vi "AlliGator Save SGL Gate Image to HDF5.vi"(6 "Compression":bool, 7 "Replace?":bool, 8 "error in (no error)":errorcluster, 9 "Image Name":string, 10 "Data":sgl[][](array[numeric]), 11 "ref in":T1 format="%.0x") -> (0 "error out":errorcluster, 3 "ref out":T1 format="%.0x")   [LabVIEW 2021, in "AlliGator Files.lvlib"]
doc: "Saves single gate image data array to HDF5 FLI Dataset file."
uses:
  AlliGator Files.lvlib
  <vilib>/addons/h5labview2/base/hid_t.ctl
  <vilib>/addons/h5labview2/base/lib_path.vi
  <vilib>/addons/h5labview2/base/H5Equery.vi
  <vilib>/addons/h5labview2/dataset/H5Dwrite.llb/H5Dwrite.xnode
  <vilib>/addons/h5labview2/props/H5P.lvlib
  <vilib>/addons/h5labview2/space/H5S.lvlib
  <vilib>/addons/h5labview2/type/H5T.lvlib
  <vilib>/addons/h5labview2/dataset/H5D.lvlib
panel:
  # "see the AlliGator License on the block diagram (Ctrl+E or Window:Show Block Diagram)"
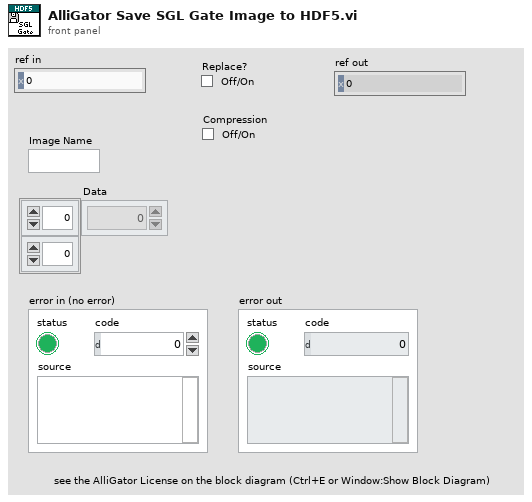
[diagram p1: front panel]
types:
  T1 = typedef "hid_t.ctl" = i64
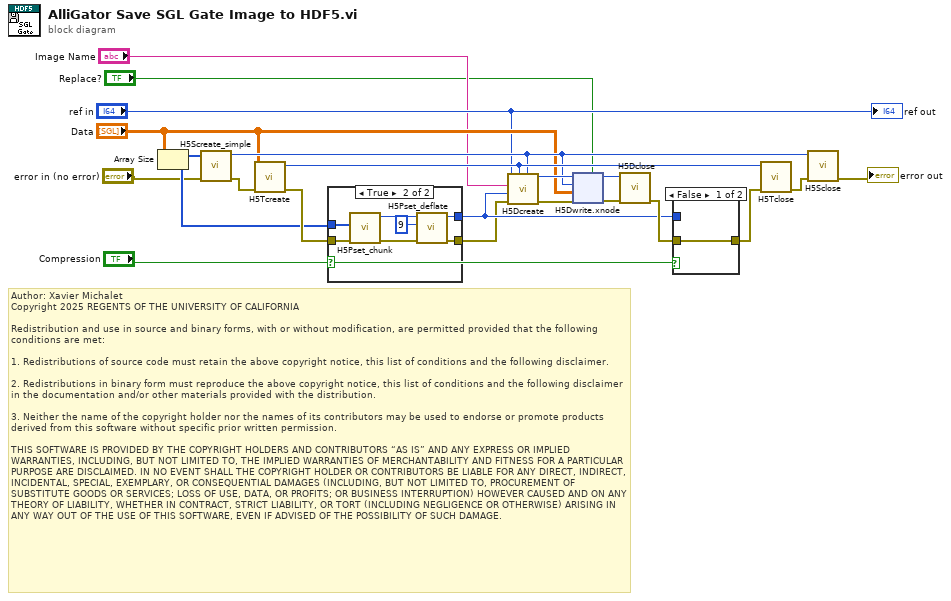
[diagram p0: block diagram]
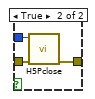
[diagram p2: hidden frame]
diagram:
  # "Author: Xavier Michalet\nCopyright 2025 REGENTS OF THE UNIVERSITY OF CALIFORNIA\n\nRedistribution and use in source and binary forms, with or without modification, are permitted provided that the following conditions are met:\n\n1. Redistributions of source code must retain the above copyright notice, this list of conditions and the following disclaimer.\n\n2. Redistributions in binary form must reproduce the above copyright notice, this list of conditions and the following disclaimer in the documentation and/or other materials provided with the distribution.\n\n3. Neither the name of the copyright holder nor the names of its contributors may be used to endorse or promote products derived from this software without specific prior written permission.\n\nTHIS SOFTWARE IS PROVIDED BY THE COPYRIGHT HOLDERS AND CONTRIBUTORS “AS IS” AND ANY EXPRESS OR IMPLIED WARRANTIES, INCLUDING, BUT NOT LIMITED TO, THE IMPLIED WARRANTIES OF MERCHANTABILITY AND FITNESS FOR A PARTICULAR PURPOSE ARE DISCLAIMED. IN NO EVENT SHALL THE COPYRIGHT HOLDER OR CONTRIBUTORS BE LIABLE FOR ANY DIRECT, INDIRECT, INCIDENTAL, SPECIAL, EXEMPLARY, OR CONSEQUENTIAL DAMAGES (INCLUDING, BUT NOT LIMITED TO, PROCUREMENT OF SUBSTITUTE GOODS OR SERVICES; LOSS OF USE, DATA, OR PROFITS; OR BUSINESS INTERRUPTION) HOWEVER CAUSED AND ON ANY THEORY OF LIABILITY, WHETHER IN CONTRACT, STRICT LIABILITY, OR TORT (INCLUDING NEGLIGENCE OR OTHERWISE) ARISING IN ANY WAY OUT OF THE USE OF THIS SOFTWARE, EVEN IF ADVISED OF THE POSSIBILITY OF SUCH DAMAGE."
  n1 = Array Size(array="Data") -> (size(s)=w8:i32[])
  n2 = call <vilib>:"H5Screate_simple.vi"("error in (no error)"="error in (no error)", "dims"=w8) -> ("error out"=w17:errorcluster, "space out"=w10:T1)  [unwired: 7 in, 1 out]
  n3 = call <vilib>:"H5Tcreate.vi"("error in (no error)"=w17, "type variant"="Data") -> ("error out"=w16:errorcluster, "type out"=w13:T1)  [unwired: 7 in, 1 out]
  n4 = case shown="True" "Compression" {
    tunnel: w16 -> [w22 w29]
    tunnel: [_ w28] -> w11
    tunnel: [w22 w24] -> w9
    tunnel: w8 -> [_ w23]
    frame False {
    }
    frame True {
      n5 = call <vilib>:"H5Pset_chunk.vi"("error in (no error)"=w29, "chunk size"=w23) -> ("error out"=w26:errorcluster, "prop out"=w27:T1)  [unwired: 8 in]
      n6 = call <vilib>:"H5Pset_deflate.vi"("error in (no error)"=w26, "level"=u8 9, "prop in"=w27) -> ("error out"=w24:errorcluster, "prop out"=w28:T1)  [unwired: 7 in]
    }
  }
  n7 = call <vilib>:"H5Dcreate.vi"("space id"=w10, "type id"=w13, "error in (no error)"=w9, "props id"=w11, "name"="Image Name", "loc in"="ref in") -> ("error out"=w15:errorcluster, "dset out"=w18:T1)  [unwired: 2 in]
  n8 = xnode "H5Dwrite.xnode"("replace? (F)"="Replace?", "error in (no error)"=w15, "data"="Data", "file space"=w10, "ref in"=w18) -> ("error out"=w21:errorcluster, "ref out"=w19:T1)  [unwired: 2 in, 1 out]
  n9 = call <vilib>:"H5Dclose.vi"("error in (no error)"=w21, "dset in"=w19) -> ("error out"=w20:errorcluster)  [unwired: 9 in]
  n10 = case shown="False" "Compression" {
    tunnel: w20 -> [w30 w33]
    tunnel: [w30 w32] -> w14
    tunnel: w11 -> [_ w31]
    frame False {
    }
    frame True {
      n11 = call <vilib>:"H5Pclose.vi"("error in (no error)"=w33, "props in"=w31) -> ("error out"=w32:errorcluster)  [unwired: 9 in]
    }
  }
  n12 = call <vilib>:"H5Tclose.vi"("error in (no error)"=w14, "type in"=w13) -> ("error out"=w12:errorcluster)  [unwired: 9 in]
  n13 = call <vilib>:"H5Sclose.vi"("error in (no error)"=w12, "space in"=w10) -> ("error out"=→"error out":errorcluster)  [unwired: 9 in]
  "ref out" <- "ref in"
